vi "Point&Path@CheckPalletLast__Parameter.vi"(1 "ParamterIn":string) -> (0 "ParamterOut":string)   [LabVIEW 2020]
panel:
  out "PointNameList":string[](array[string])
  in  "Parameter":string(combo)
  in  "PointName":string(combo)
  in  "Confirm":bool
  # "Point&Path@General $Point(,ParameterS)"
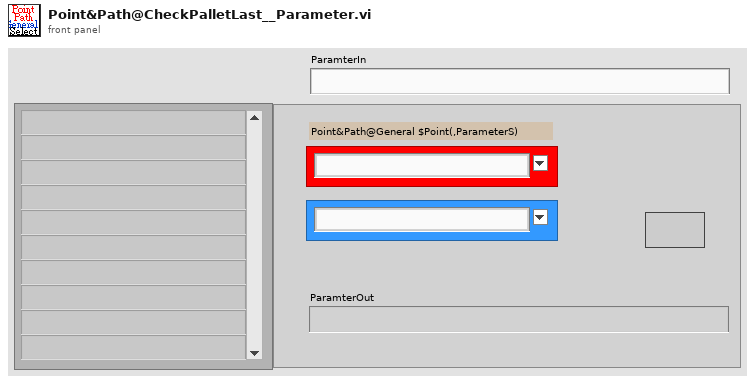
[diagram p1: front panel]
types:
  T1 = enum16{"Get", "UpdatePointS", "Init", "UpdateIndex", "GetCurrent&Index+1", "GetWithIndex", "ChkLast", "GetCurrent"}
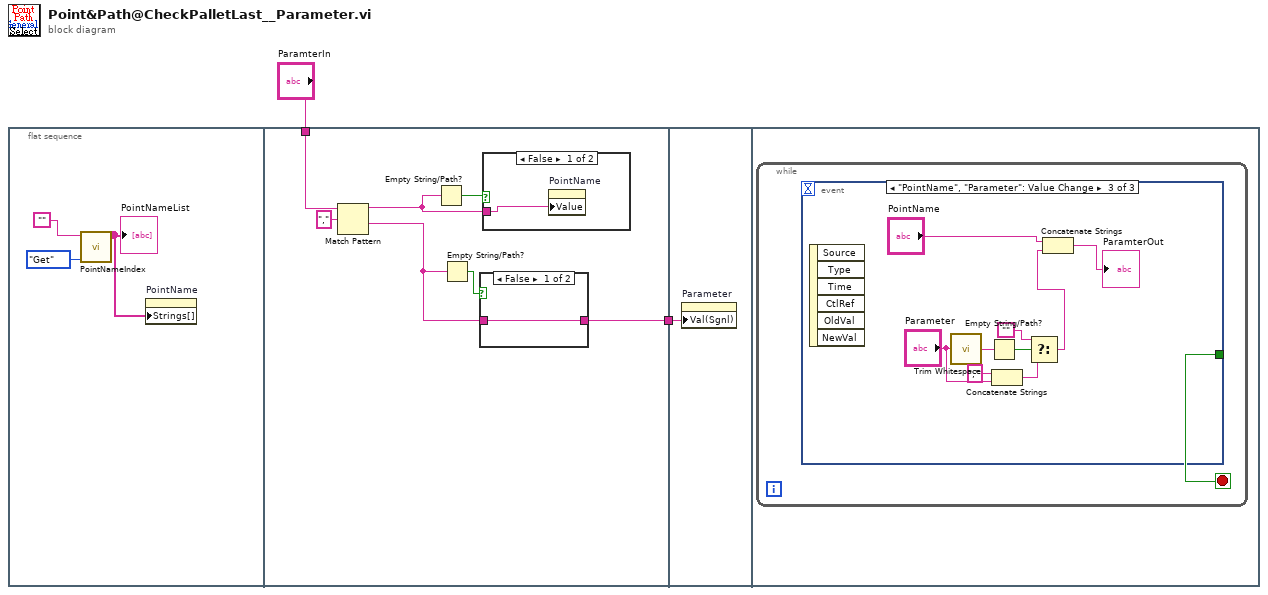
[diagram p0: block diagram]
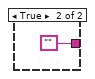
[diagram p2: hidden frame]
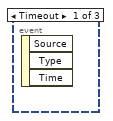
[diagram p4: hidden frame]
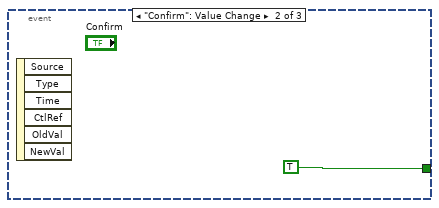
[diagram p5: hidden frame]
diagram:
  n1 = flat-sequence {
    tunnel: "ParamterIn" -> [w9]
    tunnel: [w10] -> w1
    tunnel: w1 -> [w16]
    frame #0 {
      n2 = call "PointNameIndex.vi"("OP"=T1."Get", "PointName"="") -> ("PointNameList"=w3:string[])  [unwired: 4 in, 5 out]
      "PointNameList" <- w3
      n3 = property on="PointName" class="CmbBox"("Strings[]"=w3) -> ()  [unwired: 2 in, 2 out]
    }
    frame #1 {
      n4 = Match Pattern(string=w9, regular expression="," ("search string")) -> (before substring=w6:string, after substring=w7:string)  [unwired: 1 in, 2 out]
      n5 = Empty String/Path?(string/path=w6) -> (empty?=w12:bool)
      n6 = Empty String/Path?(string/path=w7) -> (empty?=w11:bool)
      n7 = case shown="False" w11 {
        tunnel: [w13 ""] -> w10
        tunnel: w7 -> [w13 _]
        frame False {
        }
        frame True {
        }
      }
      n8 = case shown="False" w12 {
        tunnel: w6 -> [w15 _]
        frame False {
          n9 = property on="PointName" class="CmbBox"("Value"=w15) -> ()  [unwired: 2 in, 2 out]
        }
        frame True {
        }
      }
    }
    frame #2 {
      n10 = property on="Parameter" class="CmbBox"("Val(Sgnl)"=w16) -> ()  [unwired: 2 in, 2 out]
    }
    frame #3 {
      n11 = while {
        stop <- w17 stop-if-true
        n12 = event shown="[2] \"PointName\", \"Parameter\": Value Change" {
          selector: _ -> [_ _ _]
          dyn-events: _ -> [_ _ _]
          timeout: _ -> [_ _ _]
          tunnel: [_ TRUE _] -> w17
          event Timeout {
            n13 = event-data() -> ()  [unwired: 1 in, 3 out]
          }
          event "Confirm": Value Change {
            n14 = event-data() -> ()  [unwired: 1 in, 6 out]
          }
          event "PointName", "Parameter": Value Change {
            n15 = event-data() -> ()  [unwired: 1 in, 6 out]
            n16 = call <vilib>:"Trim Whitespace.vi"("string"="Parameter") -> ("trimmed string"=w22:string)  [unwired: 1 in]
            n17 = Empty String/Path?(string/path=w22) -> (empty?=w23:bool)
            n18 = Concatenate Strings("," ("string"), "Parameter") -> (w25:string)
            n19 = Select(t="", s=w23, f=w25) -> (s? t:f=w20:string)
            n20 = Concatenate Strings("PointName", w20) -> (→"ParamterOut":string)
          }
        }
      }
    }
  }
